vi "PID Controller.vi"(0 "Reference Value":dbl=30.0, 1 "Process Value":dbl format="%#_13g", 2 "Time step [s]":dbl=0.1, 3 "Previous signal":dbl, 4 "Previous error":dbl) -> (5 "Process signal":dbl, 6 "Error Term":dbl)   [LabVIEW 2023]
panel:
  in  "Propotional Gain":dbl=0.06
  in  "Integral Gain":dbl=0.3
  in  "Derivative Gain":dbl=0.3
  # "In"
  # "Out"
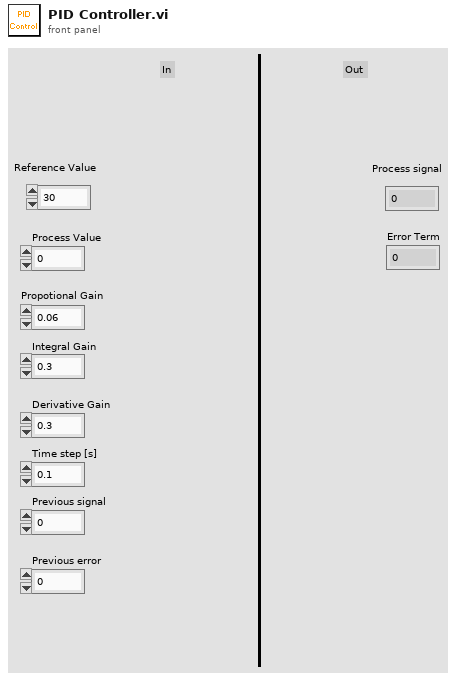
[diagram p1: front panel]
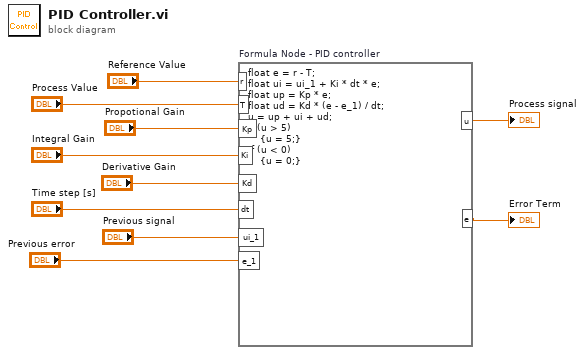
[diagram p0: block diagram]
diagram:
  n1 = formula code="float e = r - T;\nfloat ui = ui_1 + Ki * dt * e;\nfloat up = Kp * e;\nfloat ud = Kd * (e - e_1) / dt;\nu = up + ui + ud;\nif (u > 5)\n    {u = 5;}\nif (u < 0)\n    {u = 0;}" "Formula Node - PID controller"("r"="Reference Value", "T"="Process Value", "ui_1"="Previous signal", "Kp"="Propotional Gain", "Ki"="Integral Gain", "dt"="Time step [s]", "e_1"="Previous error", "Kd"="Derivative Gain") -> ("u"=→"Process signal":dbl, "e"=→"Error Term":dbl)
